vi "editor map.vi"(11 "Editor Array":u16[][](array[ring])) -> (1 "tree":bool[][](array[boolean]), 3 "fish":bool[][](array[boolean]))   [LabVIEW 2011]
uses:
  <vilib>/Utility/file.llb/Write To Spreadsheet File (I64).vi
panel:
  out "fish picture":picture
  out "badfish picture":picture
  in  "stop":bool
  out "badfish Box":u32(colorbox)=4900864
  out "fish Box":u32(colorbox)=16711680
  # "LaunchPad Game JoyStick遊戲地圖編輯器"
  # "位置"
  # "時間軸---->"
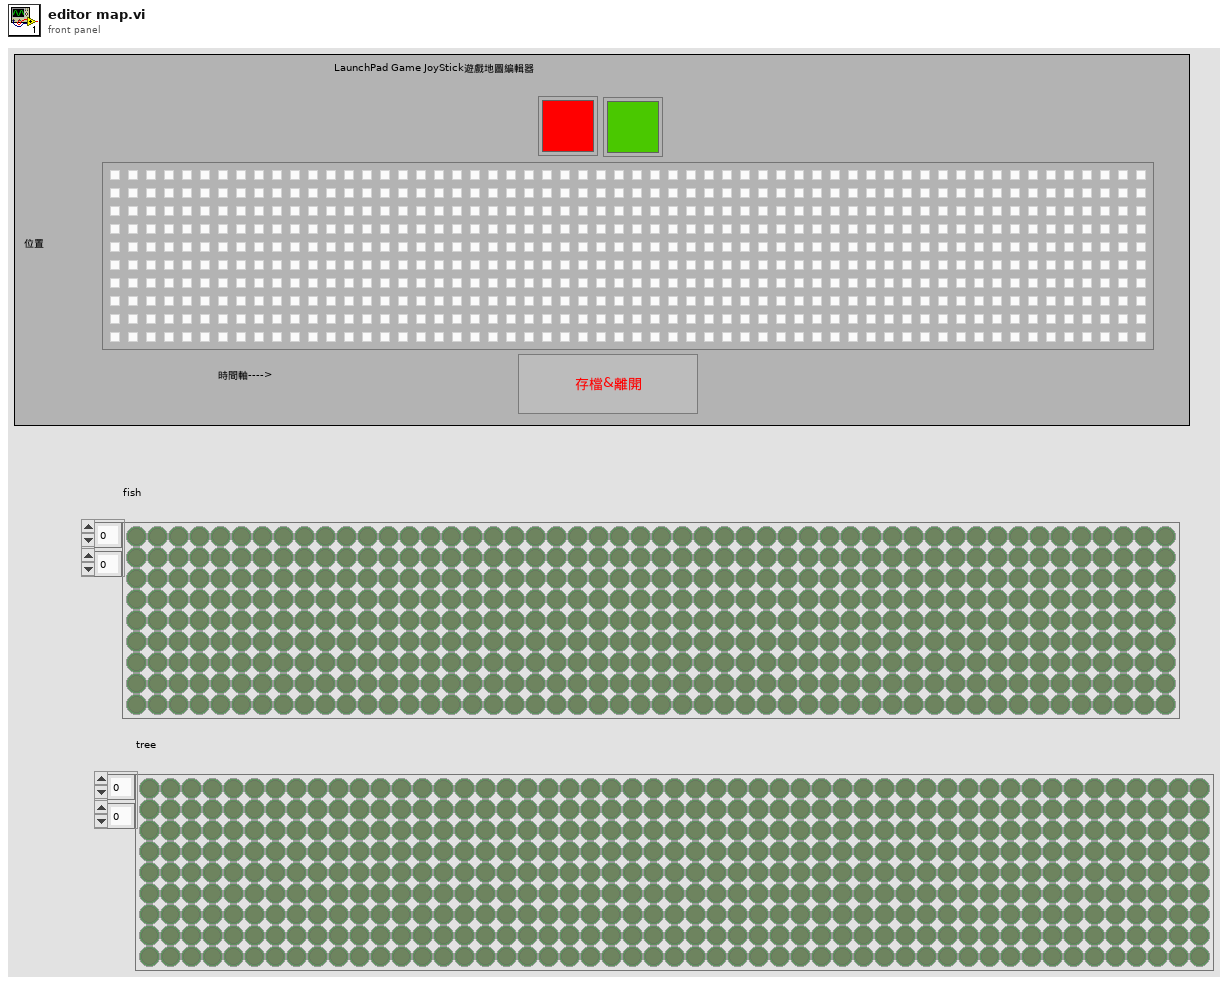
[diagram p1: front panel]
types:
  T1 = typedef "imagedata.ctl" = cluster{"image type":i32, "image depth":i32, "image":u8[], "mask":u8[], "colors":u32[], "Rectangle":cluster{"left":i16, "top":i16, "right":i16, "bottom":i16}}
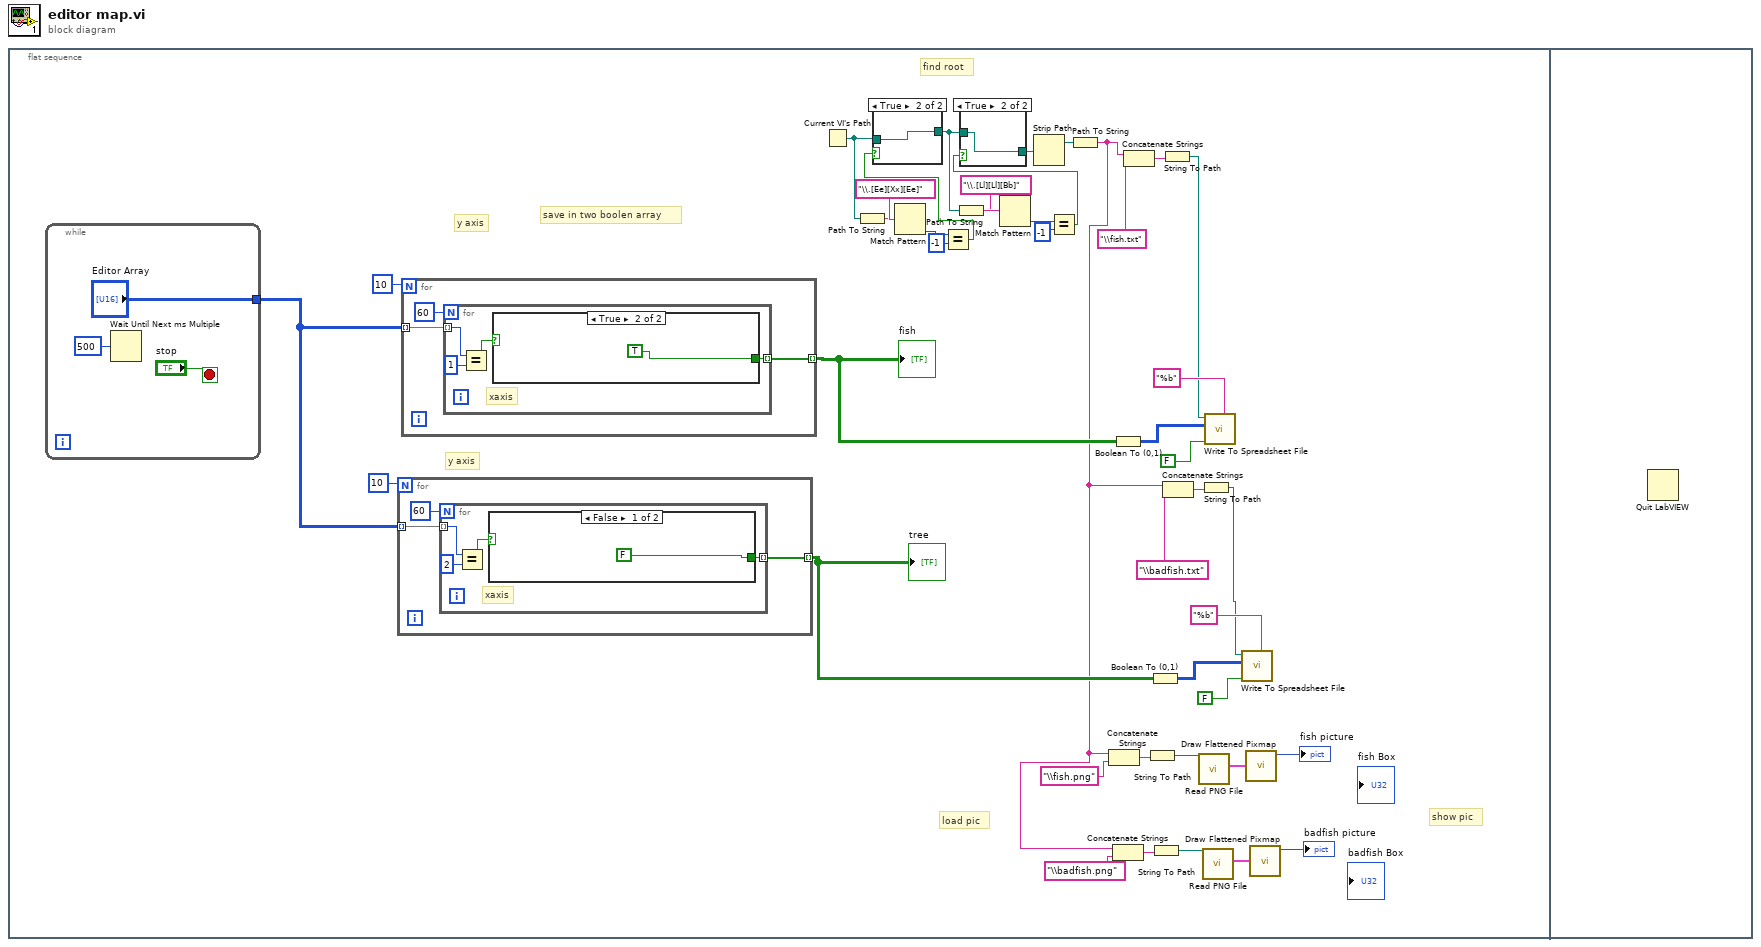
[diagram p0: block diagram]
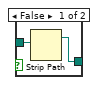
[diagram p2: hidden frame]
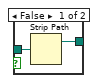
[diagram p3: hidden frame]
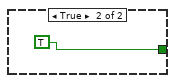
[diagram p4: hidden frame]
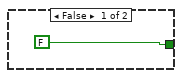
[diagram p5: hidden frame]
diagram:
  n1 = flat-sequence {
    frame #0 {
      # "save in two boolen array"
      # "show pic"
      # "load pic"
      # "find root"
      # "y axis"
      # "y axis"
      n2 = while {
        tunnel: ["Editor Array"] -> w40
        stop <- "stop" stop-if-true
        n3 = Wait Until Next ms Multiple(millisecond multiple=u32 500) -> ()  [unwired: 1 out]
      }
      n4 = for {
        N: 10 -> [_]
        tunnel: w40 -> [w54] mode=indexing
        tunnel: [w52] -> w12 mode=indexing
        n5 = for {
          N: 60 -> [_]
          tunnel: w54 -> [w55] mode=indexing
          tunnel: [w56] -> w52 mode=indexing
          # "xaxis"
          n6 = Equal?(x=w55, y=u16 2) -> (x = y?=w57:bool)
          n7 = case shown="False" w57 {
            tunnel: [FALSE TRUE] -> w56
            frame False {
            }
            frame True {
            }
          }
        }
      }
      "tree" <- w12
      n8 = for {
        N: 10 -> [_]
        tunnel: w40 -> [w63] mode=indexing
        tunnel: [w61] -> w38 mode=indexing
        n9 = for {
          N: 60 -> [_]
          tunnel: w63 -> [w64] mode=indexing
          tunnel: [w65] -> w61 mode=indexing
          # "xaxis"
          n10 = Equal?(x=w64, y=u16 1) -> (x = y?=w66:bool)
          n11 = case shown="True" w66 {
            tunnel: [FALSE TRUE] -> w65
            frame False {
            }
            frame True {
            }
          }
        }
      }
      "fish" <- w38
      n12 = Current VI's Path() -> (path=w27:path)
      n13 = Path To String(path=w27) -> (string=w26:string)
      n14 = Match Pattern(string=w26, regular expression="\\.[Ee][Xx][Ee]") -> (offset past match=w24:i32)  [unwired: 1 in, 3 out]
      n15 = Equal?(x=w24, y=-1) -> (x = y?=w36:bool)
      n16 = case shown="True" w36 {
        tunnel: [w49 w51] -> w33
        tunnel: w27 -> [w50 w51]
        frame False {
          n17 = Strip Path(path=w50) -> (stripped path=w49:path)  [unwired: 1 out]
        }
        frame True {
        }
      }
      n18 = Path To String(path=w33) -> (string=w30:string)
      n19 = Match Pattern(string=w30, regular expression="\\.[Ll][Ll][Bb]") -> (offset past match=w32:i32)  [unwired: 1 in, 3 out]
      n20 = Equal?(x=w32, y=-1) -> (x = y?=w35:bool)
      n21 = case shown="True" w35 {
        tunnel: [w46 w48] -> w34
        tunnel: w33 -> [w47 w48]
        frame False {
          n22 = Strip Path(path=w47) -> (stripped path=w46:path)  [unwired: 1 out]
        }
        frame True {
        }
      }
      n23 = Strip Path(path=w34) -> (stripped path=w23:path)  [unwired: 1 out]
      n24 = Path To String(path=w23) -> (string=w1:string)
      n25 = Concatenate Strings(w1, "\\fish.png") -> (w11:string)
      n26 = Boolean To (0,1)(Boolean=w38) -> (0, 1=w19:i16[][])
      n27 = Concatenate Strings(w1, "\\badfish.png") -> (w6:string)
      n28 = Concatenate Strings(w1, "\\fish.txt") -> (w21:string)
      n29 = String To Path(string=w11) -> (path=w9:path)
      n30 = Boolean To (0,1)(Boolean=w12) -> (0, 1=w13:i16[][])
      n31 = String To Path(string=w6) -> (path=w4:path)
      n32 = String To Path(string=w21) -> (path=w20:path)
      n33 = Concatenate Strings(w1, "\\badfish.txt") -> (w15:string)
      n34 = call <vilib>:"Read PNG File.vi"("path to PNG file"=w9) -> ("image data"=w8:T1)  [unwired: 8 in, 2 out]
      n35 = String To Path(string=w15) -> (path=w14:path)
      n36 = call <vilib>:"Read PNG File.vi"("path to PNG file"=w4) -> ("image data"=w3:T1)  [unwired: 8 in, 2 out]
      n37 = call-poly <vilib>:"Write To Spreadsheet File.vi"("format (%d)"="%b" ("format (%.3f)"), "append to file? (new file:F)"=FALSE, "2D data"=w19, "file path (dialog if empty)"=w20) -> ()  [unwired: 4 in, 1 out]
      n38 = call-poly <vilib>:"Write To Spreadsheet File.vi"("format (%d)"="%b" ("format (%.3f)"), "append to file? (new file:F)"=FALSE, "2D data"=w13, "file path (dialog if empty)"=w14) -> ()  [unwired: 4 in, 1 out]
      n39 = call <vilib>:"Draw Flattened Pixmap.vi"("image data"=w8) -> ("new picture"=→"fish picture":picture)  [unwired: 8 in]
      n40 = call <vilib>:"Draw Flattened Pixmap.vi"("image data"=w3) -> ("new picture"=→"badfish picture":picture)  [unwired: 8 in]
    }
    frame #1 {
      n41 = Quit LabVIEW() -> ()  [unwired: 1 in]
    }
  }
